vi "ModeFieldOriented.vi"(0 "Master State In":enum16{"Trap", "Climbing", "Amp", "Speaker"}(ring)) -> (1 "Robot Oriented Direction (deg)":dbl, 2 "Orientation Mode":enum16{"Robot-Oriented", "Field-Oriented"}(ring))   [LabVIEW 2023]
doc: "This VI manages whether the swerve drive is in robot-oriented or field-oriented mode, based on driver inputs, emergency overrides, and safety interlocks."
uses:
  GlobalPoseAndTargeting.vi
  GlobalDrivebase.vi
  GlobalDriverStationCommands.vi
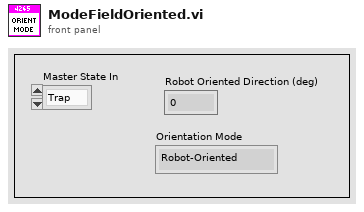
[diagram p1: front panel]
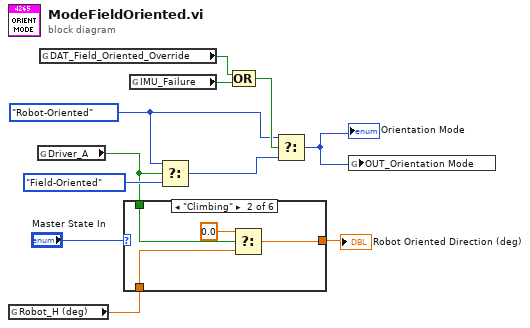
[diagram p0: block diagram]
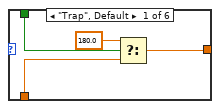
[diagram p2: hidden frame]
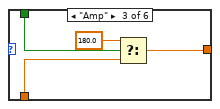
[diagram p3: hidden frame]
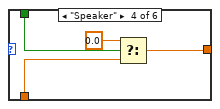
[diagram p4: hidden frame]
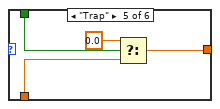
[diagram p5: hidden frame]
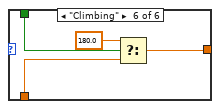
[diagram p6: hidden frame]
diagram:
  w5 = enum16{"Robot-Oriented", "Field-Oriented"}."Robot-Oriented"
  n1 = global read "GlobalPoseAndTargeting.vi" "Robot_H (deg)"() -> (w3:dbl)
  n2 = global read "GlobalDriverStationCommands.vi" "Driver_A"() -> (w2:bool)
  n3 = global read "GlobalDrivebase.vi" "DAT_Field_Oriented_Override"() -> (w9:bool)
  n4 = case shown="\"Climbing\"" "Master State In" {
    tunnel: [w14 w16 w20 w24 w28 w32] -> w4
    tunnel: w2 -> [w13 w17 w22 w25 w29 w34]
    tunnel: w3 -> [w15 w18 w21 w26 w30 w33]
    frame "Trap", Default {
      n5 = Select(t=180.0, s=w13, f=w15) -> (s? t:f=w14:dbl)
    }
    frame "Climbing" {
      n6 = Select(t=0.0, s=w17, f=w18) -> (s? t:f=w16:dbl)
    }
    frame "Amp" {
      n7 = Select(t=180.0, s=w22, f=w21) -> (s? t:f=w20:dbl)
    }
    frame "Speaker" {
      n8 = Select(t=0.0, s=w25, f=w26) -> (s? t:f=w24:dbl)
    }
    frame "Trap" {
      n9 = Select(t=0.0, s=w29, f=w30) -> (s? t:f=w28:dbl)
    }
    frame "Climbing" {
      n10 = Select(t=180.0, s=w34, f=w33) -> (s? t:f=w32:dbl)
    }
  }
  "Robot Oriented Direction (deg)" <- w4
  n11 = global read "GlobalPoseAndTargeting.vi" "IMU_Failure"() -> (w11:bool)
  n12 = Select(t=w5, s=w2, f=enum16{"Robot-Oriented", "Field-Oriented"}."Field-Oriented") -> (s? t:f=w6:enum16{"Robot-Oriented", "Field-Oriented"})
  n13 = Compound Arithmetic op=OR(w9, w11) -> (w10:bool)
  n14 = Select(t=w5, s=w10, f=w6) -> (s? t:f=w8:enum16{"Robot-Oriented", "Field-Oriented"})
  "Orientation Mode" <- w8
  n15 = global write "GlobalDrivebase.vi" "OUT_Orientation Mode"(w8) -> ()
